vi "Year2018_Q4.vi"() -> ()   [LabVIEW 2015]
panel:
  out "Original vs filtered":cluster{dbl, dbl}(graph)
  in  "stop":bool
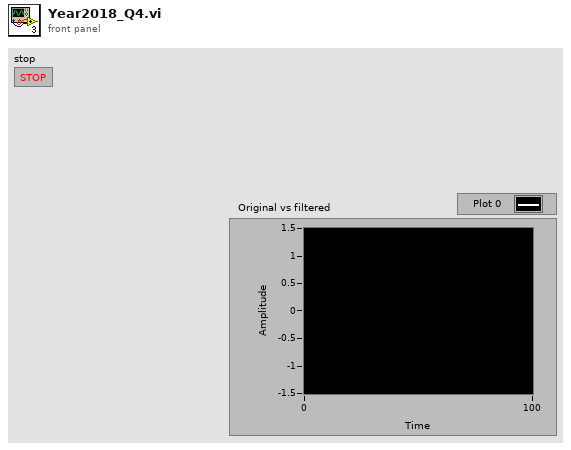
[diagram p1: front panel]
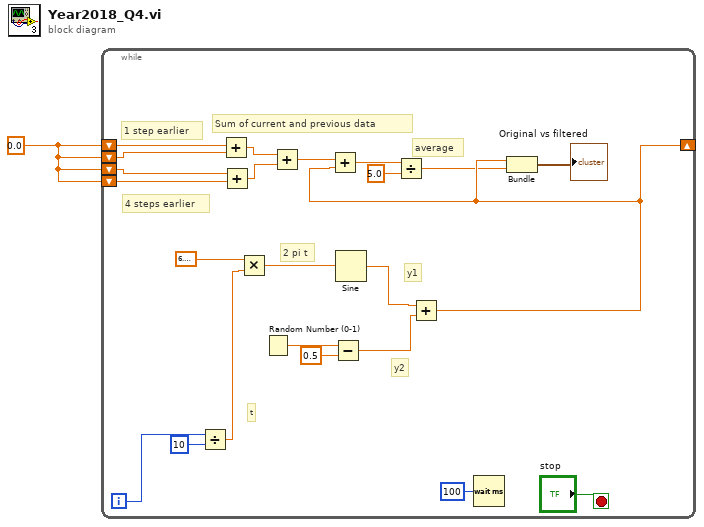
[diagram p0: block diagram]
diagram:
  w1 = 0.0
  n1 = while {
    shift-right: [w6] -> _
    shift-left: w1 -> [w13]
    shift-left: w1 -> [w12]
    shift-left: w1 -> [w11]
    shift-left: w1 -> [w10]
    i -> [w20]
    stop <- "stop" stop-if-true
    # "average"
    # "Sum of current and previous data"
    # "4 steps earlier"
    # "1 step earlier"
    # "y2"
    # "y1"
    # "2 pi t"
    # "t"
    n2 = Divide(x=w20, y=10) -> (x/y=w18:dbl)
    n3 = Add(x=w13, y=w12) -> (x+y=w9:dbl)
    n4 = Add(x=w11, y=w10) -> (x+y=w8:dbl)
    n5 = Multiply(x=6.283185307179586, y=w18) -> (x*y=w22:dbl)
    n6 = Random Number (0-1)() -> (number: 0 to 1=w17:dbl)
    n7 = Add(x=w9, y=w8) -> (x+y=w7:dbl)
    n8 = Subtract(x=w17, y=0.5) -> (x-y=w14:dbl)
    n9 = Sine(x=w22) -> (sin(x)=w15:dbl)
    n10 = Add(x=w15, y=w14) -> (x+y=w6:dbl)
    n11 = Add(x=w7, y=w6) -> (x+y=w4:dbl)
    n12 = Divide(x=w4, y=5.0) -> (x/y=w2:dbl)
    n13 = Wait (ms)(milliseconds to wait=u32 100) -> ()  [unwired: 1 out]
    n14 = Bundle(w6, w2) -> (→"Original vs filtered":cluster{dbl, dbl})  [unwired: 1 in]
  }
